vi "main_1.vi"() -> ()   [LabVIEW 2015]
uses:
  LabviewSubVI/RFConfig/RF_Config.ctl
  LabviewSubVI/RFConfig/StudentMsg.ctl
panel:
  in  "图片编码方式":enum16{"哈夫曼编码", "无编码"}(ring)=enum."无编码"
  in  "接收图片文件路径":path=path "C:/Users/liudong/Desktop/Lab15 ASK communication system1/Lab15 ASK communication system/Lab15 ASK communication system/01 TeacherVersion/matlabcode/re_tuzi.jpg"
  in  "接收语音文件路径":path=path "C:/Users/liudong/Desktop/Lab15 ASK communication system1/Lab15 ASK communication system/Lab15 ASK communication system/01 TeacherVersion/matlabcode/re_hongdou.wav"
  out "接收信号波形":dbl[](graph)
  out "发送信号波形":dbl[](graph)
  in  "循环码生成多项式":enum16{"[1,0,1,1]", "[1,1,0,1]"}(ring)=enum."[1,1,0,1]"
  out "当前帧数":i32
  out "总误码率":dbl format="%#_13g"
  out "总误码数":dbl format="%#_13g"
  out "当前帧误码率":dbl format="%#_13g"
  out "当前帧误码数":dbl format="%#_13g"
  out "当前帧CRC\n是否正确":bool[](array[boolean])
  in  "运行方式":enum16{"仿真系统", "真实系统"}(ring)
  in  "?":T1={"发射频率"=2380000000, "发射衰减"=30, "接收频率"=2380000000, "接收增益"=12, "接收通道"=enum."RxCh1", "发射通道"=enum."TxCh1"} {"接收增益" max=40 format="%.0fdB"; "接收频率" min=70000000 max=6000000000 format="%.6pHz"; "发射衰减" max=90 format="%.0fdB"; "发射频率" min=70000000 max=6000000000 format="%.6pHz"}
  in  "xsrpip":string="192.168.1.166"
  in  "pcip":string="192.168.1.180"
  in  "数据源类型":enum16{"语音", "图片", "文本"}(ring) caption="源文件格式"
  in  "汉明码编码方式":enum16{"(12,8)汉明码", "(7,4)汉明码"}(ring)
  in  "发送图片文件路径":path=path "C:/Users/liudong/Desktop/Lab15 ASK communication system1/Lab15 ASK communication system/Lab15 ASK communication system/01 TeacherVersion/matlabcode/tuzi.jpg"
  in  "发送语音文件路径":path=path "C:/Users/liudong/Desktop/Lab15 ASK communication system1/Lab15 ASK communication system/Lab15 ASK communication system/01 TeacherVersion/matlabcode/hongdou.wav"
  in  "crc位数":u16(ring)=8 items=["24"=24, "16"=16, "12"=12, "8"=8]
  out "实验学生信息":T2={"姓名"="XXX\n", "学号"="XXX", "班级"="XXX", "学校"="XXX"}
  in  "error in (no error)":errorcluster caption="错误输入（无错误）"
  out "输出文本":string
  in  "信噪比(dB)":dbl=40.0 caption="crc_num" min=-20.0 max=40.0 step=0.1 format="%#_13g"
  in  "信道编码方式":enum8{"汉明码", "循环码"}(ring)
  in  "输入文本":string="helloworld,hellochina"
  # "基于XSRP软件无线电平台的ASK数字调制通信系统"
  # "实验参数设置"
  # "实验学生信息"
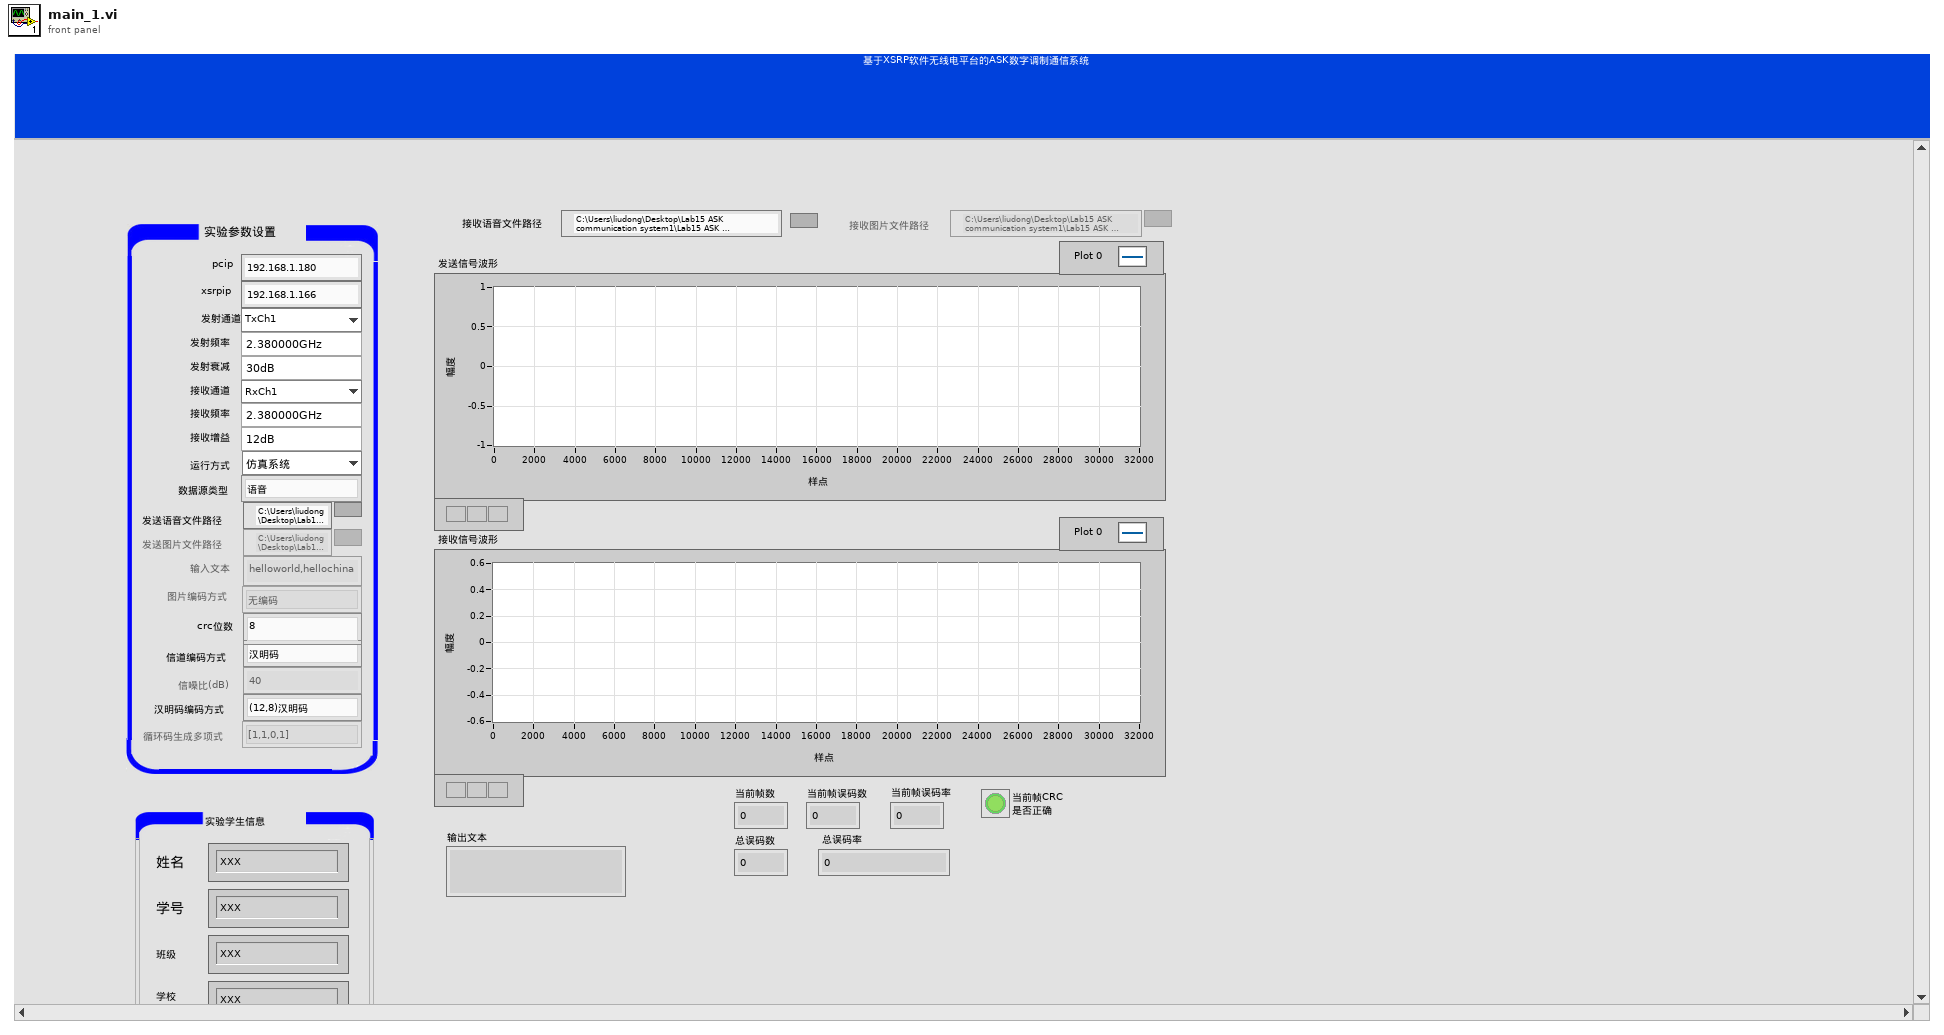
[diagram p1: front panel]
types:
  T1 = typedef "RF_Config.ctl" = cluster{"发射频率":u64, "发射衰减":u8, "接收频率":u64, "接收增益":u8, "接收通道":enum16{"RxCh1", "RxCh2"}, "发射通道":enum16{"TxCh1", "TxCh2"}}
  T2 = typedef "StudentMsg.ctl" = cluster{"姓名":string, "学号":string, "班级":string, "学校":string}
  T3 = enum8{"Enabled", "Disabled", "Disabled and Grayed Out"}
  T4 = cluster{"接收通道":enum16{"RxCh1", "RxCh2"}, "接收频率":u32, "接收增益":u8}
  T5 = cluster{"发射通道":enum16{"TxCh1", "TxCh2"}, "发射频率":u32, "发射衰减":u8}
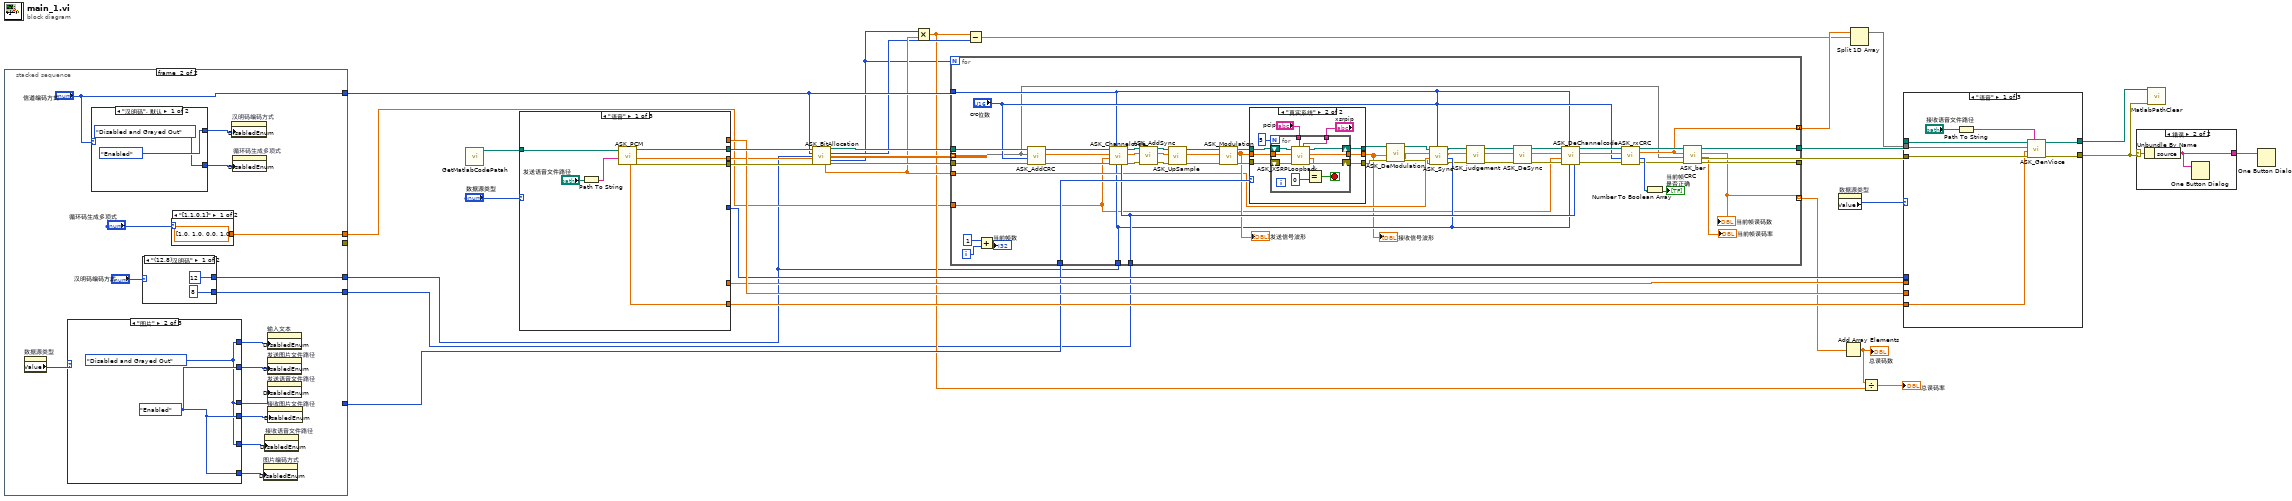
[diagram p0: block diagram]
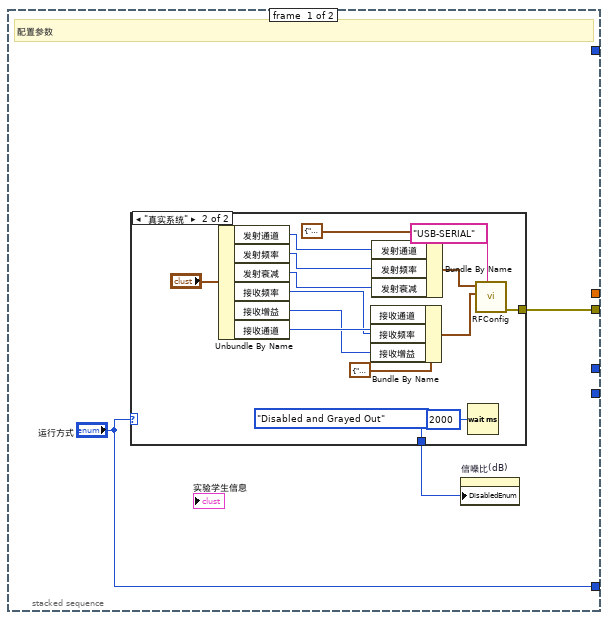
[diagram p2: hidden frame]
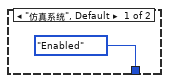
[diagram p3: hidden frame]
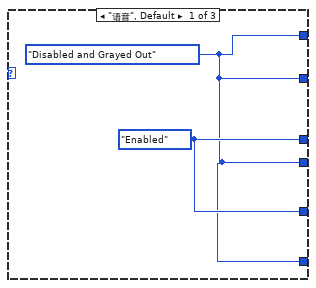
[diagram p4: hidden frame]
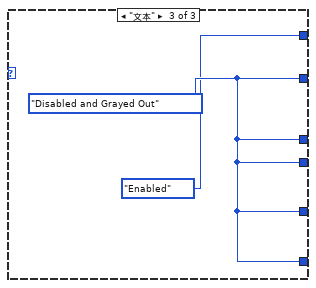
[diagram p5: hidden frame]
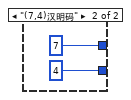
[diagram p6: hidden frame]
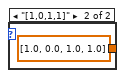
[diagram p7: hidden frame]
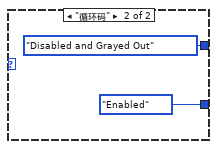
[diagram p8: hidden frame]
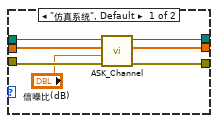
[diagram p9: hidden frame]
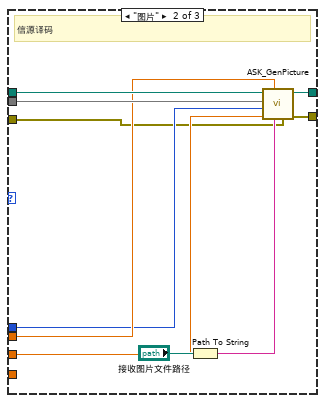
[diagram p10: hidden frame]
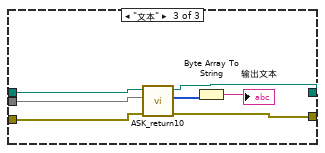
[diagram p11: hidden frame]
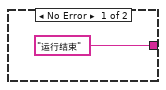
[diagram p12: hidden frame]
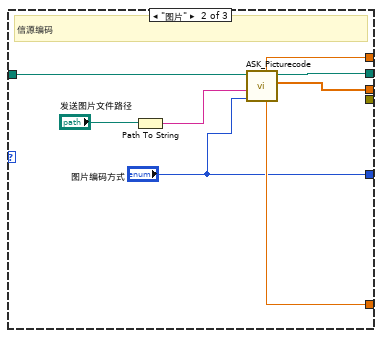
[diagram p13: hidden frame]
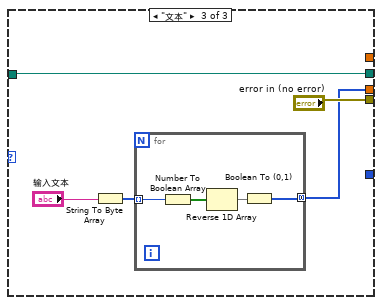
[diagram p14: hidden frame]
diagram:
  n1 = stacked-sequence {
    tunnel: [w36 _] -> _
    tunnel: ["运行方式" _] -> w10
    tunnel: [_ "信道编码方式"] -> w12
    tunnel: [_ w63] -> w4
    tunnel: [_ w61] -> w3
    tunnel: [_ w60] -> w2
    frame #0 {
      # "配置参数"
      n2 = case shown="\"真实系统\"" "运行方式" {
        tunnel: [_ w41] -> w36
        tunnel: [T3."Enabled" ("Disabled") T3."Disabled and Grayed Out" ("Disabled")] -> w34
        frame "仿真系统", Default {
        }
        frame "真实系统" {
          n3 = Unbundle By Name("?") -> ("发射通道"=w49:enum16{"TxCh1", "TxCh2"}, "发射频率"=w48:u64, "发射衰减"=w47:u8, "接收频率"=w43:u64, "接收增益"=w44:u8, "接收通道"=w45:enum16{"RxCh1", "RxCh2"})
          n4 = Bundle By Name(cluster=T4 {"接收通道"=enum."RxCh1", "接收频率"=0, "接收增益"=0} ("接收参数设置"), "接收通道"=w45, "接收频率"=w43, "接收增益"=w44) -> (w42:T4)
          n5 = Bundle By Name(cluster=T5 {"发射通道"=enum."TxCh1", "发射频率"=0, "发射衰减"=0} ("发射参数设置"), "发射通道"=w49, "发射频率"=w48, "发射衰减"=w47) -> (w51:T5)
          n6 = Wait (ms)(milliseconds to wait=u32 2000) -> ()  [unwired: 1 out]
          n7 = call "RFConfig.vi"("USB-SERIAL name"="USB-SERIAL", "接收参数设置"=w42, "发射参数设置"=w51) -> ("error out"=w41:errorcluster)  [unwired: 8 in]
        }
      }
      n8 = property on="信噪比(dB)" class="DigNum (严格)"("DisabledEnum"=w34) -> ()  [unwired: 2 in, 2 out]
    }
    frame #1 {
      n9 = property on="数据源类型" class="Enum (严格)"() -> ("Value"=w59:enum16{"语音", "图片", "文本"})  [unwired: 2 in, 2 out]
      n10 = case shown="\"图片\"" w59 {
        tunnel: [w68 w70 T3."Enabled" ("禁用")] -> w58
        tunnel: [w68 w71 w73] -> w57
        tunnel: [w68 w71 w73] -> w56
        tunnel: [w69 w70 w73] -> w55
        tunnel: [w69 w70 w73] -> w54
        tunnel: [w68 w71 w73] -> w53
        frame "语音", Default {
          w69 = T3."Enabled" ("禁用")
          w68 = T3."Disabled and Grayed Out" ("禁用")
        }
        frame "图片" {
          w71 = T3."Enabled" ("禁用")
          w70 = T3."Disabled and Grayed Out" ("禁用")
        }
        frame "文本" {
          w73 = T3."Disabled and Grayed Out" ("禁用")
        }
      }
      n11 = case shown="\"汉明码\", 默认" "信道编码方式" {
        tunnel: [T3."Disabled and Grayed Out" ("禁用") T3."Enabled" ("禁用")] -> w66
        tunnel: [T3."Enabled" ("禁用") T3."Disabled and Grayed Out" ("禁用")] -> w67
        frame "汉明码", Default {
        }
        frame "循环码" {
        }
      }
      n12 = case shown="\"(12,8)汉明码\"" "汉明码编码方式" {
        tunnel: [12 7] -> w61
        tunnel: [8 4] -> w60
        frame "(12,8)汉明码" {
        }
        frame "(7,4)汉明码" {
        }
      }
      n13 = case shown="\"[1,1,0,1]\"" "循环码生成多项式" {
        tunnel: [dbl[] [1.0, 1.0, 0.0, 1.0] dbl[] [1.0, 0.0, 1.0, 1.0] ("数值")] -> w63
        frame "[1,1,0,1]" {
        }
        frame "[1,0,1,1]" {
        }
      }
      n14 = property on="汉明码编码方式" class="Enum (严格)"("DisabledEnum"=w67) -> ()  [unwired: 2 in, 2 out]
      n15 = property on="循环码生成多项式" class="Enum (严格)"("DisabledEnum"=w66) -> ()  [unwired: 2 in, 2 out]
      n16 = property on="图片编码方式" class="Enum (严格)"("DisabledEnum"=w53) -> ()  [unwired: 2 in, 2 out]
      n17 = property on="接收语音文件路径" class="Path"("DisabledEnum"=w55) -> ()  [unwired: 2 in, 2 out]
      n18 = property on="输入文本" class="Str"("DisabledEnum"=w58) -> ()  [unwired: 2 in, 2 out]
      n19 = property on="发送图片文件路径" class="Path"("DisabledEnum"=w57) -> ()  [unwired: 2 in, 2 out]
      n20 = property on="发送语音文件路径" class="Path"("DisabledEnum"=w54) -> ()  [unwired: 2 in, 2 out]
      n21 = property on="接收图片文件路径" class="Path"("DisabledEnum"=w56) -> ()  [unwired: 2 in, 2 out]
    }
  }
  n22 = call "GetMatlabCodePatah.vi"() -> ("MatlabCodePath"=w33:path)  [unwired: 11 in]
  n23 = case shown="\"语音\"" "数据源类型" {
    tunnel: w33 -> [w90 w96 w102]
    tunnel: [w89 w95 w102] -> w30
    tunnel: [w88 w94 w99] -> w13
    tunnel: [w87 _ _] -> w31
    tunnel: [w86 _ "error in (no error)"] -> w29
    tunnel: [_ w93 _] -> w18
    tunnel: [_ w92 _] -> w17
    tunnel: [_ "图片编码方式" _] -> w14
    frame "语音" {
      n24 = Path To String(path="发送语音文件路径") -> (string=w84:string)
      n25 = call "ASK_PCM.vi"("voice_path"=w84, "PathIn"=w90) -> ("error out"=w86:errorcluster, "Origin_Bit"=w88:dbl[], "PathOut"=w89:path, "Fs"=w87:dbl)  [unwired: 6 in]
    }
    frame "图片" {
      # "信源编码"
      n26 = Path To String(path="发送图片文件路径") -> (string=w97:string)
      n27 = call "ASK_Picturecode.vi"("picture_model"="图片编码方式", "picture_path"=w97, "PathIn"=w96) -> ("Origin_Bit"=w94:dbl[], "PathOut"=w95:path, "N"=w92:dbl, "M"=w93:dbl)  [unwired: 4 in, 1 out]
    }
    frame "文本" {
      n28 = String To Byte Array(string="输入文本") -> (unsigned byte array=w100:u8[])
      n29 = for {
        tunnel: w100 -> [w107] mode=indexing
        tunnel: [w104] -> w99 mode=concatenating
        n30 = Number To Boolean Array(number=w107) -> (Boolean array=w106:bool[])
        n31 = Reverse 1D Array(array=w106) -> (reversed array=w105:bool[])
        n32 = Boolean To (0,1)(Boolean=w105) -> (0, 1=w104:i16[])
      }
    }
  }
  n33 = call "ASK_BitAllocation.vi"("PathIn"=w30, "code_model"=w12, "n"=w3, "Origin_Bit"=w13, "error in (no error)"=w29) -> ("PathOut"=w21:path, "paddingBits"=w8:i32, "FreData"=w28:dbl[][], "frame_num"=w1:i32, "bitLen"=w9:dbl, "error out"=w27:errorcluster)  [unwired: 5 in]
  n34 = Multiply(x=w1, y=w9) -> (x*y=w6:dbl)
  n35 = for {
    N: w1 -> [_]
    tunnel: w9 -> [w131]
    tunnel: w27 -> [w158]
    tunnel: [w143] -> w25 mode=concatenating
    tunnel: [w144] -> w26
    tunnel: w10 -> [w153]
    tunnel: w21 -> [w157]
    tunnel: [w146] -> w19
    tunnel: w12 -> [w128]
    tunnel: w3 -> [w130]
    tunnel: w2 -> [w152]
    tunnel: [w141] -> w11 mode=indexing
    tunnel: w4 -> [w118]
    tunnel: w28 -> [w117] mode=indexing
    i -> [w162]
    n36 = Add(x=1, y=w162) -> (x+y=→"当前帧数":i32)
    n37 = call "ASK_AddCRC.vi"("error in (no error)"=w158, "crc_num"="crc位数", "input_data"=w117, "PathIn"=w157) -> ("error out"=w155:errorcluster, "output_data"=w154:dbl[], "PathOut"=w156:path)  [unwired: 5 in]
    n38 = call "ASK_Channelcode.vi"("k"=w152, "n"=w130, "cod_mode"=w128, "error in (no error)"=w155, "生产多项式"=w118, "CRC_Bit"=w154, "PathIn"=w156) -> ("error out"=w140:errorcluster, "Channel_Bit"=w139:dbl[], "PathOut"=w138:path)  [unwired: 2 in]
    n39 = call "ASK_AddSync.vi"("error in (no error)"=w140, "Channel_Bit"=w139, "PathIn"=w138) -> ("error out"=w137:errorcluster, "data"=w136:dbl[], "PathOut"=w135:path)  [unwired: 6 in]
    n40 = call "ASK_UpSample.vi"("error in (no error)"=w137, "input_data"=w136, "PathIn"=w135) -> ("error out"=w114:errorcluster, "output_data"=w115:dbl[], "PathOut"=w116:path)  [unwired: 6 in]
    n41 = call "ASK_Modulation.vi"("error in (no error)"=w114, "input_data"=w115, "PathIn"=w116) -> ("error out"=w133:errorcluster, "out_data"=w132:cdb[], "PathOut"=w134:path)  [unwired: 6 in]
    "发送信号波形" <- w132
    n42 = case shown="\"真实系统\"" w153 {
      tunnel: w134 -> [w167 w175]
      tunnel: w132 -> [w169 w171]
      tunnel: w133 -> [w168 w176]
      tunnel: [w165 w174] -> w113
      tunnel: [w164 w173] -> w108
      tunnel: [w163 w172] -> w111
      frame "仿真系统", Default {
        n43 = call "ASK_Channel.vi"("error in (no error)"=w168, "snr"="信噪比(dB)", "txSig"=w169, "PathIn"=w167) -> ("error out"=w163:errorcluster, "rxSig"=w164:dbl[], "PathOut"=w165:path)  [unwired: 5 in]
      }
      frame "真实系统" {
        n44 = for {
          N: 5 -> [_]
          tunnel: "pcip" -> [w189]
          tunnel: "xsrpip" -> [w188]
          tunnel: [w179] -> w173
          tunnel: w171 -> [w183]
          shift-right: [w184] -> w172
          shift-left: w176 -> [w187]
          shift-right: [w185] -> w174
          shift-left: w175 -> [w186]
          stop <- w180 stop-if-true
          n45 = call "ASK_XSRPLoopback.vi"("xsrpip"=w188, "pcip"=w189, "error in (no error)"=w187, "tx_data"=w183, "PathIn"=w186) -> ("error out"=w184:errorcluster, "ERR_CODE"=w181:dbl, "rxdataIQ"=w179:cdb[], "PathOut"=w185:path)  [unwired: 3 in]
          n46 = Equal?(x=w181, y=0) -> (x = y?=w180:bool)
        }
      }
    }
    "接收信号波形" <- w108
    n47 = call "ASK_DeModulation.vi"("rx_data"=w108, "error in (no error)"=w111, "PathIn"=w113) -> ("error out"=w110:errorcluster, "PathOut"=w112:path, "data"=w109:dbl[])  [unwired: 6 in]
    n48 = call "ASK_Sync.vi"("n"=w130, "crc_num"="crc位数", "code_model"=w128, "error in (no error)"=w110, "bitLen"=w131, "input_data"=w109, "PathIn"=w112) -> ("error out"=w125:errorcluster, "output_data"=w126:dbl[], "PathOut"=w127:path)  [unwired: 2 in]
    n49 = call "ASK_judgement.vi"("error in (no error)"=w125, "input_data"=w126, "PathIn"=w127) -> ("error out"=w122:errorcluster, "judge_data"=w123:dbl[], "PathOut"=w124:path)  [unwired: 6 in]
    n50 = call "ASK_DeSync.vi"("error in (no error)"=w122, "judge_data"=w123, "PathIn"=w124) -> ("error out"=w119:errorcluster, "data1"=w120:dbl[], "PathOut"=w121:path)  [unwired: 6 in]
    n51 = call "ASK_DeChannelcode.vi"("k"=w152, "n"=w130, "cod_mode"=w128, "error in (no error)"=w119, "生产多项式"=w118, "input_data"=w120, "PathIn"=w121) -> ("error out"=w151:errorcluster, "out_data"=w150:dbl[], "PathOut"=w149:path)  [unwired: 2 in]
    n52 = call "ASK_rxCRC.vi"("error in (no error)"=w151, "crc_num"="crc位数", "input_data"=w150, "PathIn"=w149) -> ("error out"=w145:errorcluster, "CRC_flag"=w148:i32, "out_data"=w143:dbl[], "PathOut"=w147:path)  [unwired: 4 in]
    n53 = Number To Boolean Array(number=w148) -> (Boolean array=→"当前帧CRC\n是否正确":bool[])
    n54 = call "ASK_ber.vi"("error in"=w145, "rxbit"=w117, "txbit"=w143, "Path In"=w147) -> ("error out"=w144:errorcluster, "ber"=→"当前帧误码率":dbl, "errnum"=w141:dbl, "Path Out"=w146:path)  [unwired: 4 in]
    "当前帧误码数" <- w141
  }
  n55 = Subtract(x=w6, y=w8) -> (x-y=w7:dbl)
  n56 = property on="数据源类型" class="Enum (严格)"() -> ("Value"=w20:enum16{"语音", "图片", "文本"})  [unwired: 2 in, 2 out]
  n57 = Add Array Elements(numeric array=w11) -> (sum=w23:dbl)
  "总误码数" <- w23
  n58 = Split 1D Array(array=w25, index=w7) -> (first subarray=w24:dbl[])  [unwired: 1 out]
  n59 = Divide(x=w23, y=w6) -> (x/y=→"总误码率":dbl)
  n60 = case shown="\"语音\"" w20 {
    tunnel: w24 -> [w196 w205 w214]
    tunnel: [w194 w207 w212] -> w5
    tunnel: w26 -> [w197 w198 w211]
    tunnel: w31 -> [w195 _ _]
    tunnel: w19 -> [w193 w206 w210]
    tunnel: w18 -> [_ w202 _]
    tunnel: w17 -> [_ w201 _]
    tunnel: [w190 w200 w208] -> w16
    tunnel: w14 -> [_ w199 _]
    frame "语音" {
      n61 = Path To String(path="接收语音文件路径") -> (string=w191:string)
      n62 = call "ASK_GenVioce.vi"("write_filename"=w191, "error in (no error)"=w197, "sampleVal"=w195, "还原后数据"=w196, "PathIn"=w193) -> ("error out"=w194:errorcluster, "PathOut"=w190:path)  [unwired: 4 in, 1 out]
    }
    frame "图片" {
      # "信源译码"
      n63 = Path To String(path="接收图片文件路径") -> (string=w203:string)
      n64 = call "ASK_GenPicture.vi"("error in (no error)"=w198, "write_filename"=w203, "N"=w201, "M"=w202, "pic_model"=w199, "re_bits"=w205, "PathIn"=w206) -> ("error out"=w207:errorcluster, "PathOut"=w200:path)  [unwired: 3 in]
    }
    frame "文本" {
      n65 = call "ASK_return10.vi"("error in (no error)"=w211, "inputdata"=w214, "PathIn"=w210) -> ("error out"=w212:errorcluster, "outputdata"=w213:i32[], "PathOut"=w208:path)  [unwired: 6 in]
      n66 = Byte Array To String(unsigned byte array=w213) -> (string=→"输出文本":string)
    }
  }
  n67 = case shown="错误" w5 {
    selector: w5 -> [_ w217]
    tunnel: ["运行结束" ("source") w216] -> w15
    frame No Error {
    }
    frame Error {
      n68 = Unbundle By Name(w217) -> ("source"=w216:string)
      n69 = One Button Dialog(message=w216) -> ()  [unwired: 1 in, 1 out]
    }
  }
  n70 = call "MatlabPathClear.vi"("error in"=w5, "Path"=w16) -> ()  [unwired: 9 in, 1 out]
  n71 = One Button Dialog(message=w15) -> ()  [unwired: 1 in, 1 out]
